vi "scanchannel.vi"(0 "VISA resource name out":refnum<visa-resource-name>, 1 "num ch":i32, 2 "Voltage value":dbl, 3 "Init vatt value":i32, 4 "base path":path, 5 "error in":errorcluster, 6 "Integration Board IP":string, 7 "L1 Address":i32, 8 "Save test data":bool=TRUE, 9 "Ch burst":i32, 10 "Delay":i32, 11 "vclip":i32, 12 "Frequency":dbl=3000000.0, 13 "initial value":i32=50) -> (14 "VISA resource name out 2":refnum<visa-resource-name>, 15 "L1 value":i32, 19 "error out":errorcluster)   [LabVIEW 2009]
uses:
  <instrlib>/Agilent 81150/Agilent 81150.lvlib
  <vilib>/Analysis/NI_AALPro.lvlib
panel:
  out "concatenated string":string
  out "IPR value":i32
  out "Numeric":i32
  out "XY Graph 2":cluster{"Y":dbl[], "Y":dbl[]}[](graph)
  out "Data out":string="ACK\r\n"
  out "x .and. y?":bool
  out "XY Graph":cluster{"Y":dbl[], "Y":dbl[]}[](graph)
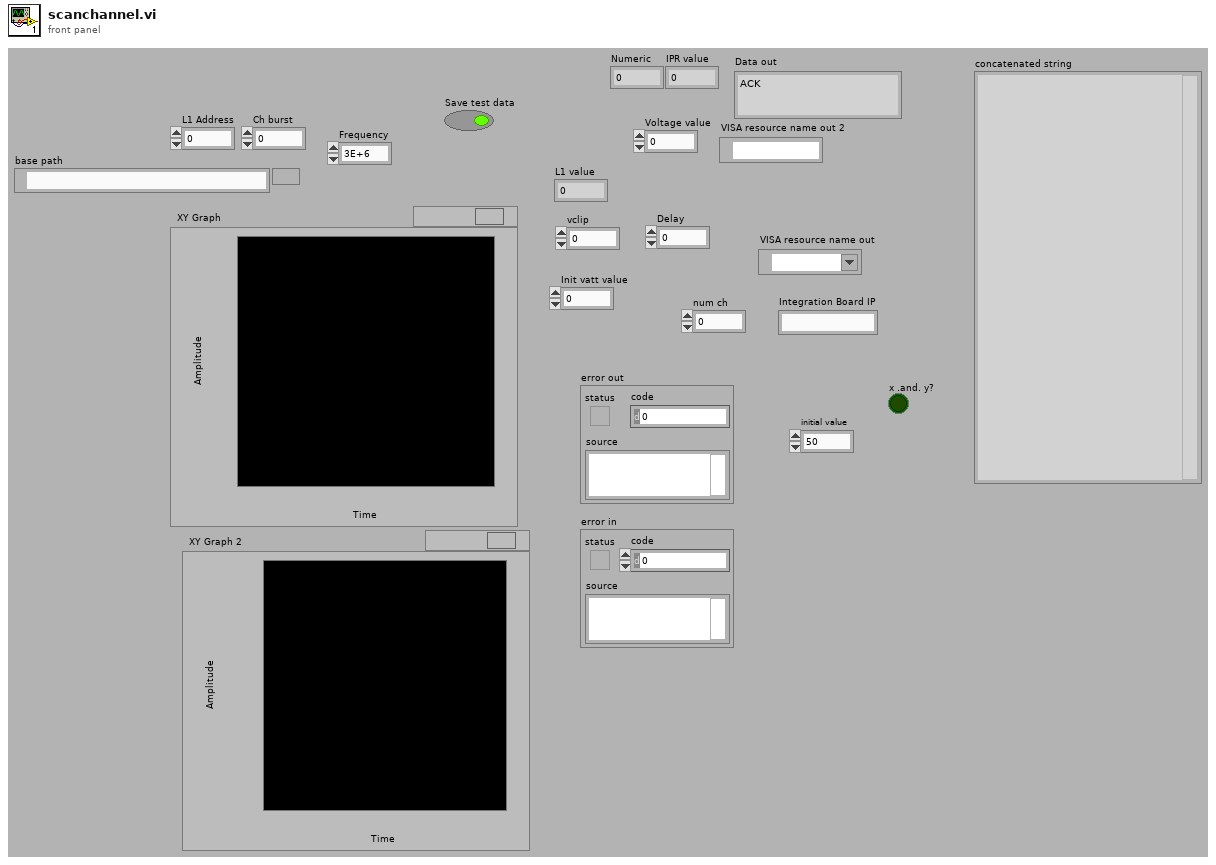
[diagram p1: front panel]
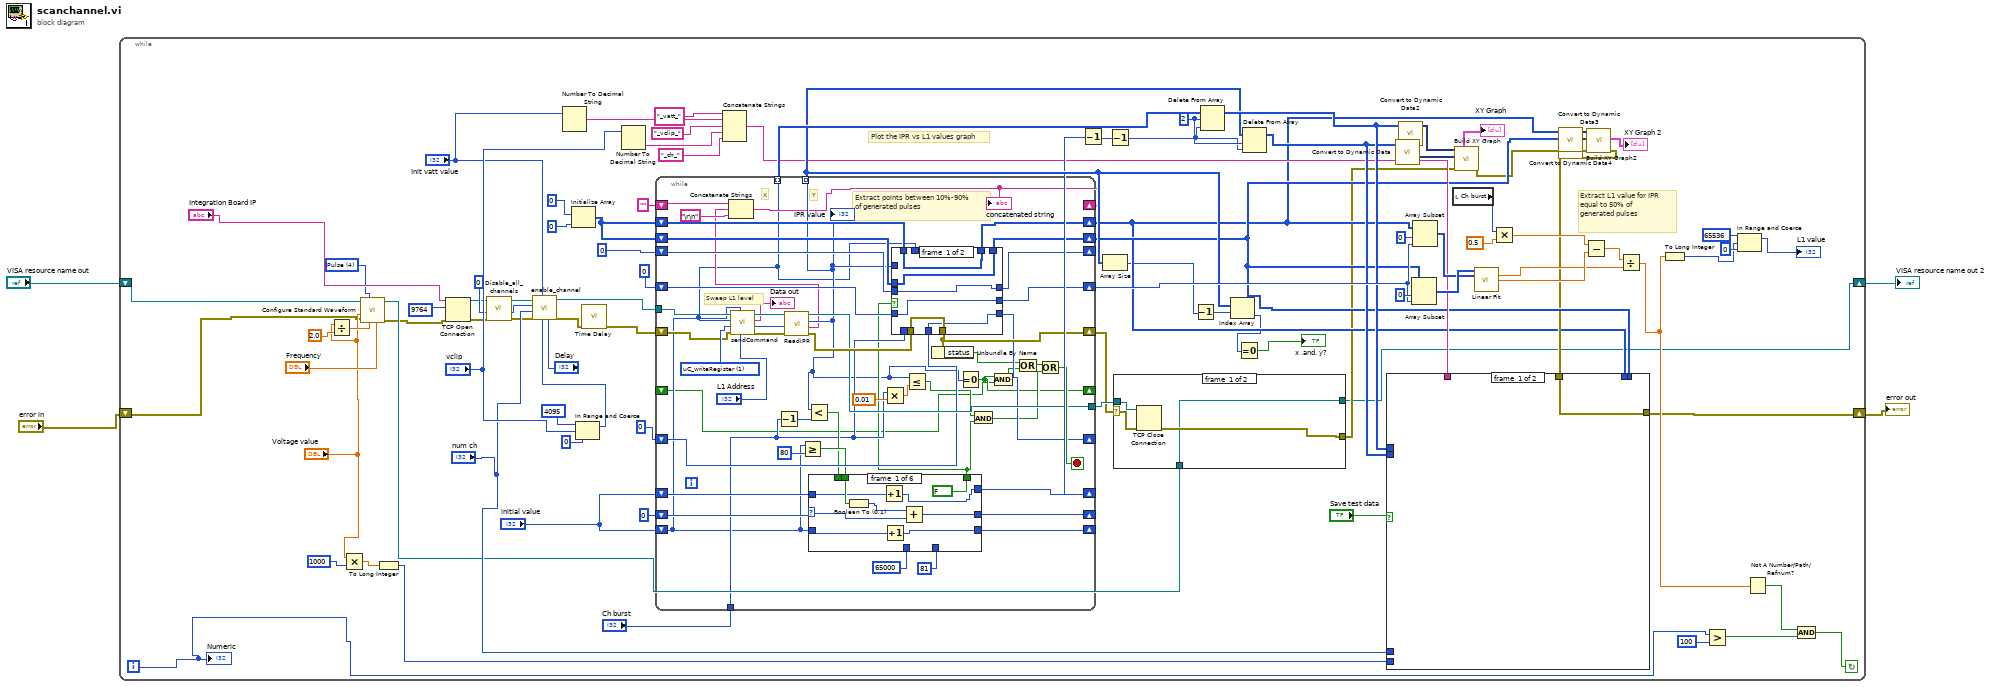
[diagram p0: block diagram]
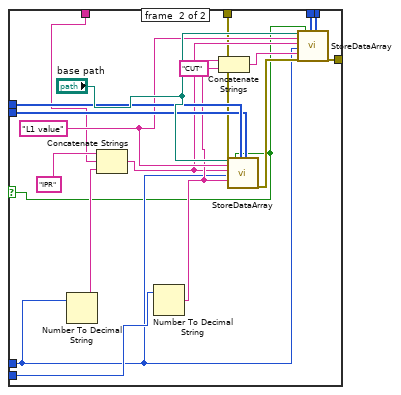
[diagram p2: hidden frame]
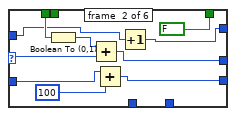
[diagram p3: hidden frame]
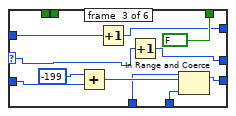
[diagram p4: hidden frame]
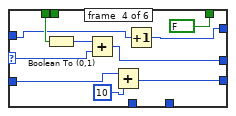
[diagram p5: hidden frame]
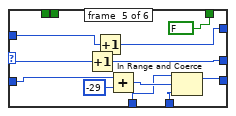
[diagram p6: hidden frame]
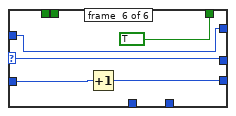
[diagram p7: hidden frame]
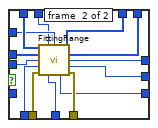
[diagram p8: hidden frame]
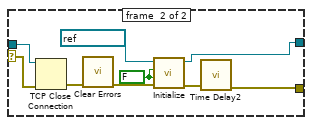
[diagram p9: hidden frame]
diagram:
  n1 = while {
    shift-right: [w17] -> w3
    shift-left: "error in" -> [w16]
    shift-right: [w13] -> w1
    shift-left: "VISA resource name out" -> [w19]
    i -> [w6]
    stop <- w7 continue-if-true
    w68 = 2 ("length")
    w96 = u16 4 items=["Sine", "Square", "Ramp Up", "Ramp Down", "Pulse", "Noise", "DC"] ("Waveform (0: Sine)")
    # "Extract L1 value for IPR equal to 50% of generated pulses"
    # "Plot the IPR vs L1 values graph"
    n2 = Divide(x="Voltage value", y=2.0) -> (x/y=w94:dbl)
    n3 = Multiply(x="Voltage value", y=1000) -> (x*y=w90:dbl)
    n4 = call <instrlib>:"Configure Standard Waveform.vi"("Frequency (1000.0 Hz)"="Frequency", "DC Offset (0.0 Volts)"=w94, "Waveform (0: Sine)"=w96, "error in (no error)"=w16, "Amplitude (1.0 Vpp)"="Voltage value", "VISA resource name"=w19) -> ("error out"=w12:errorcluster, "VISA resource name out"=w14:refnum<visa-resource-name>)  [unwired: 4 in]
    n5 = To Long Integer(number=w90) -> (32bit integer=w89:i32)
    n6 = TCP Open Connection(address="Integration Board IP", remote port or service name=u16 9764, error in (no error)=w12) -> (connection ID=w37:refnum<k5>, error out=w38:errorcluster)  [unwired: 2 in]
    n7 = call "Disable_all_channels.vi"("error in"=w38, "id_in"=0, "connection ID"=w37) -> ("error out"=w42:errorcluster, "id_out"=w39:i32, "connection ID out"=w41:refnum<k5>)  [unwired: 6 in]
    n8 = Number To Decimal String(number="Init vatt value") -> (decimal integer string=w65:string)  [unwired: 1 in]
    n9 = Initialize Array(0 ("element"), 0 ("dimension size")) -> (w46:i32[])
    n10 = In Range and Coerce(upper limit=4095, x="vclip", lower limit=0) -> (coerced(x)=w27:i32)  [unwired: 1 out]
    n11 = call "enable_channel.vi"("Delay"="Delay", "V clip"=w27, "V att"="Init vatt value", "error in"=w42, "Channel"="num ch", "id_in"=w39, "connection ID"=w41) -> ("error out"=w10:errorcluster, "connection ID out"=w40:refnum<k5>)  [unwired: 2 in, 1 out]
    n12 = call "Time Delay"("error in (no error)"=w10) -> ("error out"=w11:errorcluster)  [unwired: 10 in]
    n13 = Number To Decimal String(number="vclip") -> (decimal integer string=w64:string)  [unwired: 1 in]
    n14 = while {
      tunnel: [w133] -> w71 mode=indexing
      tunnel: [w126] -> w73 mode=indexing
      shift-right: [w167] -> w53
      shift-left: w46 -> [w165]
      shift-right: [w166] -> w58
      shift-left: w46 -> [w164]
      shift-right: [w160] -> w15
      shift-left: w11 -> [w151]
      shift-right: [w162] -> _
      shift-left: 0 ("Array Pointer out") -> [w163]
      tunnel: w40 -> [w152]
      tunnel: [w153] -> w30
      shift-right: [w161] -> w82
      shift-left: 0 ("N_Array Elements") -> [w150]
      shift-right: [w148] -> _
      shift-left: 0 ("State machine") -> [w149]
      tunnel: "Ch burst" -> [w138]
      shift-right: [w144] -> _
      shift-left: 0 -> [w146]
      shift-right: [w143] -> _
      shift-left: "initial value" -> [w126]
      shift-right: [w141] -> w69
      shift-left: "initial value" -> [w140]
      shift-right: [w130] -> _
      shift-left: "" -> [w131]
      shift-right: [w123] -> _
      shift-left: _ -> [w122]
      stop <- w159 stop-if-true
      w158 = u16 1 items=["sendCommand"=9, "FPGA_writeRegister"=3, "FPGA_readRegister"=2, "uC_writeRegister"=1, "uC_readRegister"=0] ("Action")
      # "Extract points between 10%-90% of generated pulses"
      # "Sweep L1 level"
      # "Y"
      # "X"
      n15 = call "sendCommand.vi"("Address"="L1 Address", "Data"=w126, "error in"=w151, "Action"=w158, "id_in"=w126, "connection ID"=w152) -> ("error out"=w157:errorcluster, "id_out"=w129:i32, "Data out"=→"Data out":string, "connection ID out"=w156:refnum<k5>)  [unwired: 1 in, 1 out]
      n16 = Decrement(x=w138) -> (x-1=w139:i32)
      n17 = call "ReadIPR.vi"("error in"=w157, "id_in"=w129, "connection ID"=w156) -> ("error out"=w155:errorcluster, "Data out"=w127:string, "IPR value"=w133:i32, "connection ID out"=w153:refnum<k5>)  [unwired: 4 in, 1 out]
      "IPR value" <- w133
      n18 = Concatenate Strings(w131, w127, "\r\n") -> (w130:string)
      "concatenated string" <- w130
      n19 = Greater Or Equal?(x=w126, y=80) -> (x >= y?=w145:bool)
      n20 = Less?(x=w133, y=w139) -> (x < y?=w142:bool)
      n21 = case shown="0, Default" w146 {
        selector: w146 -> [w176 w186 w199 w204 w217 w223]
        tunnel: w145 -> [w178 _ _ _ _ _]
        tunnel: [w175 w185 w195 w202 w216 w223] -> w144
        tunnel: [w173 w182 w191 w207 w212 w224] -> w143
        tunnel: w126 -> [w174 w184 w198 w208 w219 w225]
        tunnel: w142 -> [_ w188 _ w205 _ _]
        tunnel: [FALSE FALSE FALSE FALSE FALSE TRUE] -> w137
        tunnel: [w171 w180 w194 w201 w215 w221] -> w141
        tunnel: w140 -> [w170 w179 w193 w200 w218 w221]
        tunnel: 81 ("lower limit") -> [_ _ w190 _ w211 _]
        tunnel: 65000 ("upper limit") -> [_ _ w189 _ w210 _]
        frame #0 {
          n22 = Boolean To (0,1)(Boolean=w178) -> (0, 1=w177:i16)
          n23 = Increment(x=w170) -> (x+1=w171:i32)
          n24 = Increment(x=w174) -> (x+1=w173:i32)
          n25 = Add(x=w177, y=w176) -> (x+y=w175:i32)
        }
        frame #1 {
          n26 = Boolean To (0,1)(Boolean=w188) -> (0, 1=w187:i16)
          n27 = Add(x=w187, y=w186) -> (x+y=w185:i32)
          n28 = Add(x=w184, y=100) -> (x+y=w182:i32)
          n29 = Increment(x=w179) -> (x+1=w180:i32)
        }
        frame #2 {
          n30 = Add(x=-199, y=w198) -> (x+y=w192:i32)
          n31 = Increment(x=w193) -> (x+1=w194:i32)
          n32 = Increment(x=w199) -> (x+1=w195:i32)
          n33 = In Range and Coerce(upper limit=w189, x=w192, lower limit=w190) -> (coerced(x)=w191:i32)  [unwired: 1 out]
        }
        frame #3 {
          n34 = Boolean To (0,1)(Boolean=w205) -> (0, 1=w203:i16)
          n35 = Add(x=w203, y=w204) -> (x+y=w202:i32)
          n36 = Add(x=w208, y=10) -> (x+y=w207:i32)
          n37 = Increment(x=w200) -> (x+1=w201:i32)
        }
        frame #4 {
          n38 = Increment(x=w217) -> (x+1=w216:i32)
          n39 = Increment(x=w218) -> (x+1=w215:i32)
          n40 = Add(x=w219, y=-29 ("x")) -> (x+y=w213:i32)
          n41 = In Range and Coerce(upper limit=w210, x=w213, lower limit=w211) -> (coerced(x)=w212:i32)  [unwired: 1 out]
        }
        frame #5 {
          n42 = Increment(x=w225) -> (x+1=w224:i32)
        }
      }
      n43 = Multiply(x=w138, y=0.01) -> (x*y=w168:dbl)
      n44 = case shown="False" w137 {
        tunnel: [w231 w245] -> w167
        tunnel: [w230 w244] -> w166
        tunnel: w165 -> [w231 w243]
        tunnel: w164 -> [w230 w242]
        tunnel: w163 -> [w228 w241]
        tunnel: [w228 w240] -> w162
        tunnel: [w227 w239] -> w161
        tunnel: w138 -> [_ w238]
        tunnel: [w229 w237] -> w160
        tunnel: w155 -> [w229 w236]
        tunnel: w133 -> [_ w235]
        tunnel: w126 -> [_ w234]
        tunnel: w150 -> [w227 _]
        tunnel: w149 -> [w226 w233]
        tunnel: [w226 w232] -> w148
        frame #0 {
        }
        frame #1 {
          n45 = call "FittingRange.vi"("Array in (X)"=w243, "L0 DAC"=w234, "IPR"=w235, "Array in (Y)"=w242, "Array Pointer in"=w241, "Cycles Burst"=w238, "error in"=w236, "State machine"=w233) -> ("Array out (X)"=w245:i32[], "Array out (Y)"=w244:i32[], "Array Pointer out"=w240:i32, "N_Array Elements"=w239:i32, "State machine"=w232:i32, "error out"=w237:errorcluster)  [unwired: 2 in]
        }
      }
      n46 = Less Or Equal?(x=w133, y=w168) -> (x <= y?=w136:bool)
      n47 = Unbundle By Name(w160) -> ("status"=w134:bool)
      n48 = Equal To 0?(x=w133) -> (x = 0?=w123:bool)
      n49 = And(x=w136, y=w137) -> (x .and. y?=w135:bool)
      n50 = And(x=w123, y=w122) -> (x .and. y?=w124:bool)
      n51 = Or(x=w134, y=w124) -> (x .or. y?=w125:bool)
      n52 = Or(x=w125, y=w135) -> (x .or. y?=w159:bool)
    }
    n53 = Concatenate Strings("_vatt_" ("string"), w65, "_vclip_" ("string"), w64, "_ch_" ("string")) -> (w60:string)
    n54 = Decrement(x=w69) -> (x-1=w66:i32)
    n55 = Array Size(array=w71) -> (size(s)=w33:i32)
    n56 = Decrement(x=w66) -> (x-1=w67:i32)
    n57 = case shown="No Error" w15 {
      selector: w15 -> [w248 w257]
      tunnel: w30 -> [w249 w258]
      tunnel: [w247 w252] -> w24
      tunnel: w14 -> [w246 _]
      tunnel: [w246 w253] -> w13
      frame #0 {
        n58 = TCP Close Connection(connection ID=w249, error in (no error)=w248) -> (error out=w247:errorcluster)  [unwired: 1 in, 1 out]
      }
      frame #1 {
        w254 = FALSE ("Reset (True)")
        n59 = TCP Close Connection(connection ID=w258, error in (no error)=w257) -> (error out=w251:errorcluster)  [unwired: 1 in, 1 out]
        n60 = call <vilib>:"Clear Errors.vi"("error in (no error)"=w251) -> ("error out"=w255:errorcluster)  [unwired: 6 in]
        n61 = call <instrlib>:"Initialize.vi"("error in (no error)"=w255, "Reset (True)"=w254, "ID Query (True)"=w254, "VISA resource name"=refnum<visa-resource-name> "81160A") -> ("error out"=w256:errorcluster, "VISA resource name out"=w253:refnum<visa-resource-name>)  [unwired: 6 in]
        n62 = call "Time Delay2"("error in (no error)"=w256) -> ("error out"=w252:errorcluster)  [unwired: 10 in]
      }
    }
    n63 = Decrement(x=w33) -> (x-1=w34:i32)
    n64 = Delete From Array(array=w73, length=w68, index=w67) -> (array with subset deleted=w72:i32[])  [unwired: 1 out]
    n65 = Index Array(array=w71, index=w34) -> (element=w31:i32)
    n66 = Equal To 0?(x=w31) -> (x = 0?=→"x .and. y?":bool)
    n67 = Delete From Array(array=w71, length=w68, index=w67) -> (array with subset deleted=w70:i32[])  [unwired: 1 out]
    n68 = call "Convert to Dynamic Data"("Array"=w70) -> ("Dynamic Data Type"=w86:dynamicdata)  [unwired: 3 in]
    n69 = call "Convert to Dynamic Data2"("Array"=w72) -> ("Dynamic Data Type"=w85:dynamicdata)  [unwired: 3 in]
    n70 = Array Subset(array=w58, index=0, length=w82) -> (w81:i32[])
    n71 = Array Subset(array=w53, index=0, length=w82) -> (w80:i32[])
    n72 = local read "Ch burst"() -> (w74:i32)
    n73 = call "Build XY Graph"("error in (no error)"=w24, "Y Input"=w86, "X Input"=w85) -> ("error out"=w56:errorcluster, "XY Graph"=→"XY Graph":cluster{"Y":dbl[], "Y":dbl[]}[])  [unwired: 7 in]
    n74 = call <vilib>:"Linear Fit.vi"("Y"=w81, "X"=w80) -> ("slope"=w75:dbl, "intercept"=w77:dbl)  [unwired: 9 in, 3 out]
    n75 = Multiply(x=w74, y=0.5) -> (x*y=w78:dbl)
    n76 = call "Convert to Dynamic Data3"("Array"=w53) -> ("Dynamic Data Type"=w59:dynamicdata)  [unwired: 3 in]
    n77 = call "Convert to Dynamic Data4"("Array"=w58) -> ("Dynamic Data Type"=w57:dynamicdata)  [unwired: 3 in]
    n78 = Subtract(x=w78, y=w77) -> (x-y=w76:dbl)
    n79 = call "Build XY Graph2"("error in (no error)"=w56, "Y Input"=w57, "X Input"=w59) -> ("error out"=w55:errorcluster, "XY Graph"=→"XY Graph 2":cluster{"Y":dbl[], "Y":dbl[]}[])  [unwired: 7 in]
    n80 = case shown="False" "Save test data" {
      selector: "Save test data" -> [_ w101]
      tunnel: [w100 w119] -> w17
      tunnel: w89 -> [_ w118]
      tunnel: w72 -> [_ w113]
      tunnel: w70 -> [_ w112]
      tunnel: w60 -> [_ w107]
      tunnel: w58 -> [_ w105]
      tunnel: w55 -> [w100 w104]
      tunnel: w53 -> [_ w103]
      tunnel: "num ch" -> [_ w102]
      frame #0 {
      }
      frame #1 {
        w111 = "L1 value" ("X Signal Name")
        n81 = Number To Decimal String(number=w102) -> (decimal integer string=w106:string)  [unwired: 1 in]
        n82 = Concatenate Strings("IPR" ("Y Signal Name"), w107, w106) -> (w108:string)
        n83 = Number To Decimal String(number=w118) -> (decimal integer string=w110:string)  [unwired: 1 in]
        n84 = Concatenate Strings(w110, "CUT" ("string")) -> (w116:string)
        n85 = call "StoreDataArray.vi"("Base path"="base path", "X Signal Name"=w111, "Y Signal Name"=w108, "Channel number"=w102, "Si"=w110, "error in"=w104, "Save test data"=w101, "X Array"=w113, "Y Array"=w112) -> ("error out"=w117:errorcluster)  [unwired: 10 in]
        n86 = call "StoreDataArray.vi"("Base path"="base path", "X Signal Name"=w111, "Y Signal Name"=w108, "Channel number"=w102, "Si"=w116, "error in"=w117, "Save test data"=w101, "X Array"=w103, "Y Array"=w105) -> ("error out"=w119:errorcluster)  [unwired: 10 in]
      }
    }
    n87 = Divide(x=w76, y=w75) -> (x/y=w21:dbl)
    n88 = To Long Integer(number=w21) -> (32bit integer=w88:i32)
    n89 = Greater?(x=w6, y=100) -> (0:w9:bool)
    n90 = In Range and Coerce(upper limit=65536, x=w88, lower limit=0) -> (coerced(x)=→"L1 value":i32)  [unwired: 1 out]
    n91 = Not A Number/Path/Refnum?(number/path/refnum=w21) -> (NaN/Path/Refnum?=w8:bool)
    n92 = And(x=w8, y=w9) -> (x .and. y?=w7:bool)
    "Numeric" <- w6
  }
  "error out" <- w3
  "VISA resource name out 2" <- w1
